vi "subGenerateDGMLReferenceString.vi"(9 "References":set{string}(c389), 11 "Source":string) -> (1 "Links":T1)   [LabVIEW 2020, in "DefaultExtensions.lvlib" / "CGrapherDGML.lvclass"]
uses:
  CGrapherDGML.lvclass
  obj/Addons/LabVIEWItem.lvlibp/LabVIEWItem/CLabVIEWItem/ConnectionSet.ctl
  obj/Addons/LabVIEWItem.lvlibp/LabVIEWItem/CLabVIEWItem/CLabVIEWItem.lvclass
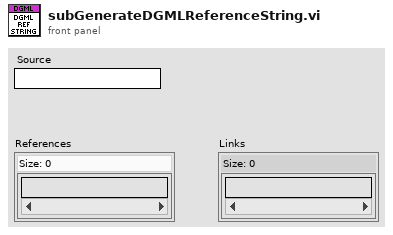
[diagram p1: front panel]
types:
  T1 = typedef "LabVIEWItem.lvlibp/CLabVIEWItem.lvclass/ConnectionSet.ctl" = set{string}
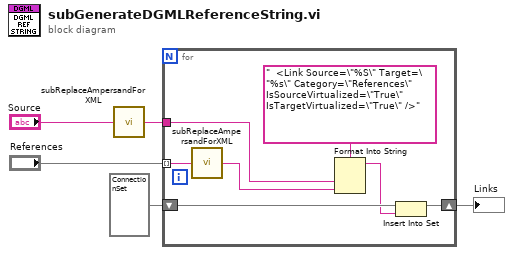
[diagram p0: block diagram]
diagram:
  n1 = call "subReplaceAmpersandForXML.vi"("String"="Source") -> ("result string"=w4:string)
  n2 = for {
    tunnel: "References" -> [w12] mode=indexing
    tunnel: w4 -> [w10]
    shift-right: [w8] -> w1
    shift-left: T1 {} ("Nodes") -> [w9]
    n3 = call "subReplaceAmpersandForXML.vi"("String"=w12) -> ("result string"=w6:string)
    n4 = Format Into String(format string="  <Link Source=\"%S\" Target=\"%s\" Category=\"References\" IsSourceVirtualized=\"True\" IsTargetVirtualized=\"True\" />", w10, w6) -> (resulting string=w7:string)  [unwired: 2 in, 1 out]
    n5 = Insert Into Set(10:w7, 11:w9) -> (3:w8:T1)  [unwired: 1 out]
  }
  "Links" <- w1
